vi "PH_AxisGUI_NF.panel.vi"(0 "object ref":refnum<vi>, 5 "error in (no error)":errorcluster) -> (19 "error out":errorcluster)   [LabVIEW 2014, in "PH_AxisGUI_NF.lvlib"]
doc: "By this VI a ross relais can be monitored and switched. \n\nThe indicators \"CLOSED\", \"OPEN\" and \"SWITCH STATE\" show the value of the Beckhoff-Tag: blue indicates bad tag status reference problems, darkgreen false and lightgreen on. If everything is working fine, \"CLOSED\" and \"SWITCH STATE\" should show the same value, while \"OPEN\" has the opposite value. \n\nThe oval button switches the ross relais. It should be in the same state as the \"SWITCH STATE\" indicator. \n\n\"EXIT\" closes the front panel (GUI), while \"Delete Instance\" disconnects and removes the instance from the PCS.\n\nThis VI has no machine safety relevant logig: there is neither a check of internal conclict nor with other objects, for example conflict with other ross relais. Therefore it must be handled with care and should be operated by well educated operators only. It is forseen exclusively for direct operating and testing of the system. \n\nLicense Agreement for this software:\n\nCopyright (C)\nGesellschaft für Schwerionenforschung, GSI\nPlanckstr. 1\n64291 Darmstadt\nGermany\n\nContact: D.Beck@gsi.de \n\nThis program is free software; you can redistribute it and/or modify it under the terms of the GNU General Public License as published by the Free Software Foundation; either version 2 of the license, or (at your option) any later version.\n\nThis program is distributed in the hope that it will be useful, but WITHOUT ANYW ARRANTY; without even the implied warranty of MERCHANTABILITY or FITNESS FOR A PARTICULAR PURPOSE. See the GNU General License for more details (http://www.gnu.org).\n\nGesellschaft für Schwerionenforschung, GSI\nPlanckstr. 1, 64291 Darmstadt, Germany\nFor all questions and ideas contact: M.Richter@gsi.de, H.Brand@gsi.de or D.Beck@gsi.de.\nLast update: 18-DEC-2002"
uses:
  PH_AxisGUI_NF.lvlib
  CSMotion/NF87XX/NF87XX.lvlib
  PH_Common/PH_Common.lvlib
  PH_Class/PH_Class.lvlib
panel:
  in  "Goal":string="0"
  in  "Go":bool
  in  "Reset":bool
  out "Position":i32
  out "Instance Status":u32(colorbox)
  in  "Slide 2":i32(slide) scale=-8.0..8.0
  in  "Slide 1":i32(slide) scale=-8.0..8.0
  in  "Slide 0":i32(slide) scale=-8.0..8.0
  in  "Emergeny Stop":bool
  in  "Delete":bool
  # "PCS"
  # "3.40"
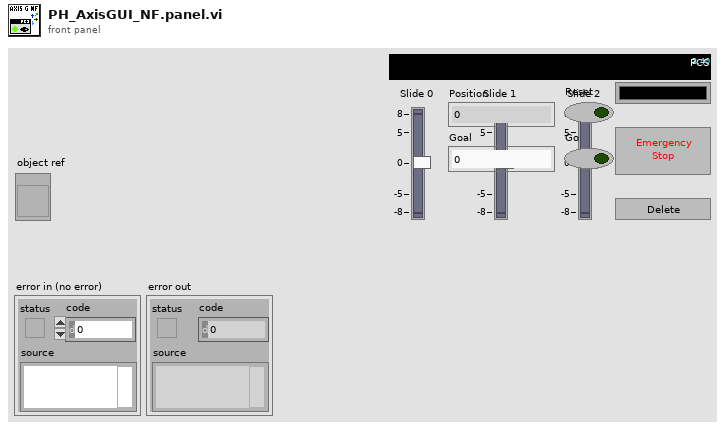
[diagram p1: front panel]
types:
  T1 = typedef "PH_AxisGUI_NF.lvlib/PH_AxisGUI_NF.i attribute.ctl" = cluster{"GUI Refs":cluster{"Delete":refnum<vi>, "Slide 0":refnum<vi>, "Slide 1":refnum<vi>, "Slide 2":refnum<vi>, "Instance Status":refnum<vi>, "Position":refnum<vi>, "Reset":refnum<vi>, "Goal":refnum<vi>, "Go":refnum<vi>}, "Instance":string, "Name Axis 0":string, "Name Axis 1":string, "Name Axis 2":string, "System":string, "Driver Type":T2, "Offset":i32, "Goal":i32}
  T2 = typedef "NF87XX.lvlib/NF87XX.driver Type.ctl" = enum16{"not defined", "3-ch open loop drv", "1-ch closed loop drv"}
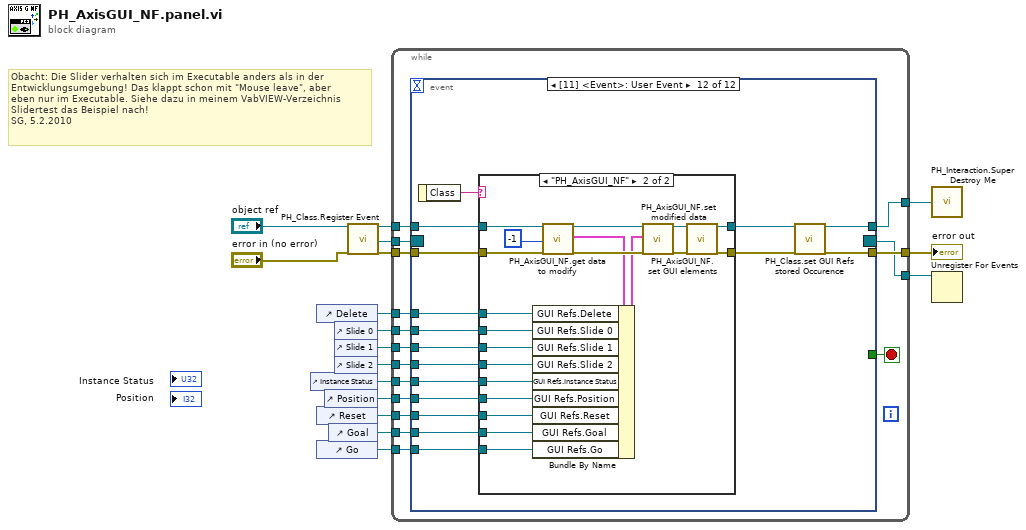
[diagram p0: block diagram]
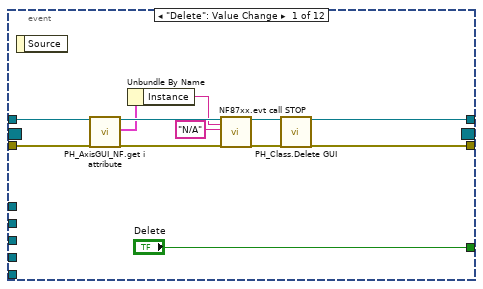
[diagram p2: hidden frame]
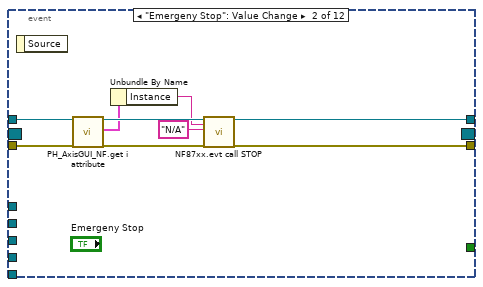
[diagram p3: hidden frame]
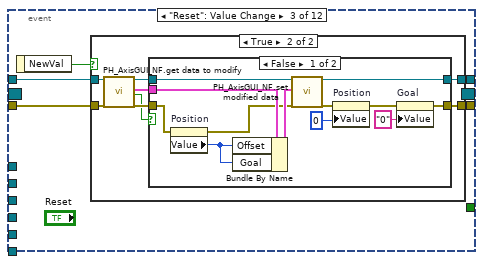
[diagram p4: hidden frame]
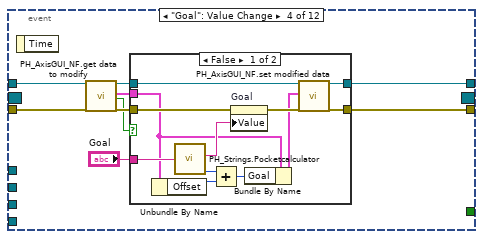
[diagram p7: hidden frame]
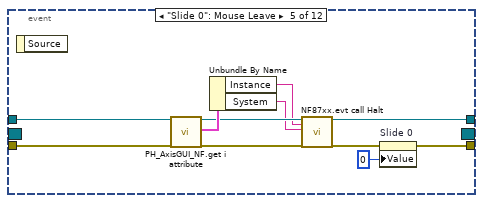
[diagram p9: hidden frame]
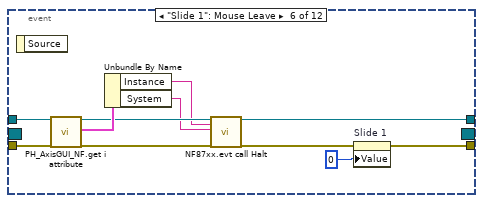
[diagram p10: hidden frame]
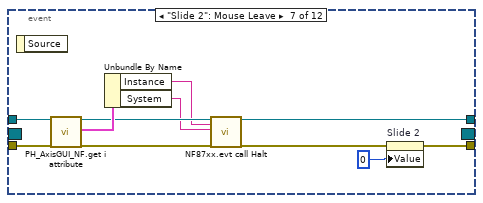
[diagram p11: hidden frame]
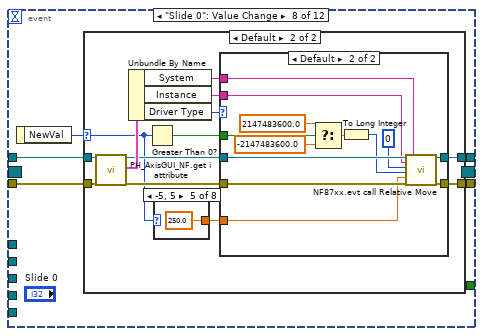
[diagram p12: hidden frame]
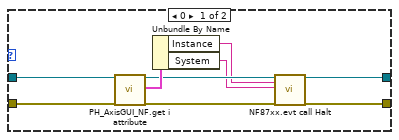
[diagram p13: hidden frame]
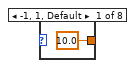
[diagram p14: hidden frame]
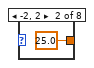
[diagram p15: hidden frame]
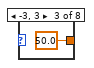
[diagram p16: hidden frame]
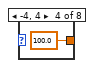
[diagram p17: hidden frame]
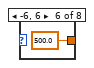
[diagram p18: hidden frame]
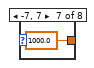
[diagram p19: hidden frame]
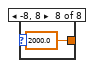
[diagram p20: hidden frame]
diagram:
  # "Obacht: Die Slider verhalten sich im Executable anders als in der\nEntwicklungsumgebung! Das klappt schon mit \"Mouse leave\", aber \neben nur im Executable. Siehe dazu in meinem VabVIEW-Verzeichnis\nSlidertest das Beispiel nach!\nSG, 5.2.2010"
  n1 = control-ref of="Instance Status"() -> (w7:refnum<vi>)
  n2 = control-ref of="Delete"() -> (w11:refnum<vi>)
  n3 = control-ref of="Reset"() -> (w5:refnum<vi>)
  n4 = control-ref of="Go"() -> (w3:refnum<vi>)
  n5 = control-ref of="Position"() -> (w6:refnum<vi>)
  n6 = control-ref of="Goal"() -> (w4:refnum<vi>)
  n7 = control-ref of="Slide 0"() -> (w10:refnum<vi>)
  n8 = control-ref of="Slide 1"() -> (w9:refnum<vi>)
  n9 = control-ref of="Slide 2"() -> (w8:refnum<vi>)
  n10 = call "PH_Class.Register Event.vi"("i ref in"="object ref", "error in (no error)"="error in (no error)") -> ("i ref out"=w15:refnum<vi>, "Event Registration Refnum"=w13:refnum<event-registration>, "error out"=w14:errorcluster)  [unwired: 15 in]
  n11 = while {
    tunnel: w15 -> [w30]
    tunnel: [w29] -> w17
    tunnel: w14 -> [w32]
    tunnel: [w31] -> w16
    tunnel: w13 -> [w28]
    tunnel: [w27] -> w12
    tunnel: w11 -> [w26]
    tunnel: w10 -> [w25]
    tunnel: w9 -> [w24]
    tunnel: w8 -> [w23]
    tunnel: w7 -> [w22]
    tunnel: w6 -> [w21]
    tunnel: w5 -> [w20]
    tunnel: w4 -> [w19]
    tunnel: w3 -> [w18]
    stop <- w33 stop-if-true
    n12 = event shown="[11] <Event>: User Event" {
      selector: w28 -> [_ _ _ _ _ _ _ _ _ _ _ _]
      dyn-events: [_ _ _ _ _ _ _ _ _ _ _ _] -> w27
      timeout: _ -> [_ _ _ _ _ _ _ _ _ _ _ _]
      tunnel: ["Delete" _ _ _ _ _ _ _ _ _ _ _] -> w33
      tunnel: w30 -> [w39 w50 w57 w87 w112 w126 w137 w142 w200 w249 w299 w357]
      tunnel: w32 -> [w37 w52 w56 w90 w110 w124 w135 w144 w199 w250 w300 w356]
      tunnel: [w34 w54 w59 w88 w116 w120 w131 w143 w197 w247 w298 w359] -> w31
      tunnel: [w35 w53 w58 w86 w113 w127 w138 w141 w198 w246 w297 w360] -> w29
      tunnel: w26 -> [_ _ _ _ _ _ _ _ _ _ _ w353]
      tunnel: w25 -> [_ _ _ _ _ _ _ _ _ _ _ w352]
      tunnel: w24 -> [_ _ _ _ _ _ _ _ _ _ _ w351]
      tunnel: w23 -> [_ _ _ _ _ _ _ _ _ _ _ w350]
      tunnel: w22 -> [_ _ _ _ _ _ _ _ _ _ _ w349]
      tunnel: w21 -> [_ _ _ _ _ _ _ _ _ _ _ w348]
      tunnel: w20 -> [_ _ _ _ _ _ _ _ _ _ _ w347]
      tunnel: w19 -> [_ _ _ _ _ _ _ _ _ _ _ w346]
      tunnel: w18 -> [_ _ _ _ _ _ _ _ _ _ _ w345]
      event "Delete": Value Change {
        n13 = event-data() -> ()  [unwired: 1 in, 1 out]
        n14 = call "PH_AxisGUI_NF.get i attribute.vi"("i ref in"=w39, "error in (no error)"=w37) -> ("i ref out"=w43:refnum<vi>, "i attribute"=w42:T1, "error out"=w44:errorcluster)  [unwired: 15 in]
        n15 = Unbundle By Name(w42) -> ("Instance"=w41:string)
        n16 = call "NF87xx.evt call STOP.vi"("i ref in"=w43, "Instance"=w41, "System (N/A)"="N/A", "error in (no error)"=w44) -> ("i ref out"=w38:refnum<vi>, "error out"=w36:errorcluster)  [unwired: 14 in]
        n17 = call "PH_Class.Delete GUI.vi"("VI in"=w38, "error in (no error)"=w36) -> ("VI out"=w35:refnum<vi>, "error out"=w34:errorcluster)  [unwired: 16 in]
      }
      event "Emergeny Stop": Value Change {
        n18 = event-data() -> ()  [unwired: 1 in, 1 out]
        n19 = call "PH_AxisGUI_NF.get i attribute.vi"("i ref in"=w50, "error in (no error)"=w52) -> ("i ref out"=w49:refnum<vi>, "i attribute"=w48:T1, "error out"=w51:errorcluster)  [unwired: 15 in]
        n20 = Unbundle By Name(w48) -> ("Instance"=w47:string)
        n21 = call "NF87xx.evt call STOP.vi"("i ref in"=w49, "Instance"=w47, "System (N/A)"="N/A", "error in (no error)"=w51) -> ("i ref out"=w53:refnum<vi>, "error out"=w54:errorcluster)  [unwired: 14 in]
      }
      event "Reset": Value Change {
        n22 = event-data() -> ("NewVal"=w55:bool)  [unwired: 1 in]
        n23 = case shown="True" w55 {
          tunnel: [w60 w69] -> w59
          tunnel: [w61 w68] -> w58
          tunnel: w57 -> [w61 w67]
          tunnel: w56 -> [w60 w65]
          frame False {
          }
          frame True {
            n24 = call "PH_AxisGUI_NF.get data to modify.vi"("i ref in"=w67, "error in (no error)"=w65) -> ("i ref out"=w66:refnum<vi>, "i attribute"=w62:T1, "timed out"=w63:bool, "error out"=w64:errorcluster)  [unwired: 14 in]
            n25 = case shown="False" w63 {
              tunnel: [w72 w82] -> w69
              tunnel: [w81 w83] -> w68
              tunnel: w66 -> [w80 w83]
              tunnel: w64 -> [w77 w82]
              tunnel: w62 -> [w79 _]
              frame False {
                n26 = property on="Position" class="DigNum (strict)"(error in=w77) -> (error out=w76:errorcluster, "Value"=w70:i32)  [unwired: 1 in, 1 out]
                n27 = Bundle By Name(cluster=w79, "Offset"=w70, "Goal"=w70) -> (w78:T1)
                n28 = call "PH_AxisGUI_NF.set modified data.vi"("i ref in"=w80, "i attribute"=w78, "error in (no error)"=w76) -> ("i ref out"=w81:refnum<vi>, "error out"=w75:errorcluster)  [unwired: 15 in]
                n29 = property on="Position" class="DigNum (strict)"(error in=w75, "Value"=0 ("Position")) -> (error out=w73:errorcluster)  [unwired: 1 in, 1 out]
                n30 = property on="Goal" class="Str"(error in=w73, "Value"="0" ("Goal")) -> (error out=w72:errorcluster)  [unwired: 1 in, 1 out]
              }
              frame True {
              }
            }
          }
        }
      }
      event "Goal": Value Change {
        n31 = event-data() -> ()  [unwired: 1 in, 1 out]
        n32 = call "PH_AxisGUI_NF.get data to modify.vi"("i ref in"=w87, "error in (no error)"=w90) -> ("i ref out"=w91:refnum<vi>, "i attribute"=w85:T1, "timed out"=w84:bool, "error out"=w89:errorcluster)  [unwired: 14 in]
        n33 = case shown="False" w84 {
          tunnel: "Goal" -> [w104 _]
          tunnel: w91 -> [w102 w106]
          tunnel: w89 -> [w101 w105]
          tunnel: [w99 w105] -> w88
          tunnel: [w98 w106] -> w86
          tunnel: w85 -> [w96 _]
          frame False {
            n34 = Unbundle By Name(w96) -> ("Offset"=w94:i32)
            n35 = call "PH_Strings.Pocketcalculator.vi"("Input"=w104) -> ("String Integer"=w103:string, "Integer"=w95:i32)  [unwired: 2 out]
            n36 = Add(x=w95, y=w94) -> (x+y=w93:i32)
            n37 = property on="Goal" class="Str"(error in=w101, "Value"=w103) -> (error out=w100:errorcluster)  [unwired: 1 in, 1 out]
            n38 = Bundle By Name(cluster=w96, "Goal"=w93) -> (w97:T1)
            n39 = call "PH_AxisGUI_NF.set modified data.vi"("i ref in"=w102, "i attribute"=w97, "error in (no error)"=w100) -> ("i ref out"=w98:refnum<vi>, "error out"=w99:errorcluster)  [unwired: 15 in]
          }
          frame True {
          }
        }
      }
      event "Slide 0": Mouse Leave {
        n40 = event-data() -> ()  [unwired: 1 in, 1 out]
        n41 = call "PH_AxisGUI_NF.get i attribute.vi"("i ref in"=w112, "error in (no error)"=w110) -> ("i ref out"=w111:refnum<vi>, "i attribute"=w115:T1, "error out"=w109:errorcluster)  [unwired: 15 in]
        n42 = Unbundle By Name(w115) -> ("Instance"=w108:string, "System"=w107:string)
        n43 = call "NF87xx.evt call Halt.vi"("i ref in"=w111, "Instance"=w108, "System"=w107, "error in (no error)"=w109) -> ("i ref out"=w113:refnum<vi>, "error out"=w114:errorcluster)  [unwired: 14 in]
        n44 = property on="Slide 0" class="Slide (strict)"(error in=w114, "Value"=0 ("Slide 0")) -> (error out=w116:errorcluster)  [unwired: 1 in, 1 out]
      }
      event "Slide 1": Mouse Leave {
        n45 = event-data() -> ()  [unwired: 1 in, 1 out]
        n46 = call "PH_AxisGUI_NF.get i attribute.vi"("i ref in"=w126, "error in (no error)"=w124) -> ("i ref out"=w125:refnum<vi>, "i attribute"=w128:T1, "error out"=w123:errorcluster)  [unwired: 15 in]
        n47 = Unbundle By Name(w128) -> ("Instance"=w122:string, "System"=w118:string)
        n48 = call "NF87xx.evt call Halt.vi"("i ref in"=w125, "Instance"=w122, "System"=w118, "error in (no error)"=w123) -> ("i ref out"=w127:refnum<vi>, "error out"=w121:errorcluster)  [unwired: 14 in]
        n49 = property on="Slide 1" class="Slide (strict)"(error in=w121, "Value"=0 ("Slide 0")) -> (error out=w120:errorcluster)  [unwired: 1 in, 1 out]
      }
      event "Slide 2": Mouse Leave {
        n50 = event-data() -> ()  [unwired: 1 in, 1 out]
        n51 = call "PH_AxisGUI_NF.get i attribute.vi"("i ref in"=w137, "error in (no error)"=w135) -> ("i ref out"=w136:refnum<vi>, "i attribute"=w139:T1, "error out"=w134:errorcluster)  [unwired: 15 in]
        n52 = Unbundle By Name(w139) -> ("Instance"=w133:string, "System"=w129:string)
        n53 = call "NF87xx.evt call Halt.vi"("i ref in"=w136, "Instance"=w133, "System"=w129, "error in (no error)"=w134) -> ("i ref out"=w138:refnum<vi>, "error out"=w132:errorcluster)  [unwired: 14 in]
        n54 = property on="Slide 2" class="Slide (strict)"(error in=w132, "Value"=0 ("Slide 0")) -> (error out=w131:errorcluster)  [unwired: 1 in, 1 out]
      }
      event "Slide 0": Value Change {
        n55 = event-data() -> ("NewVal"=w140:i32)  [unwired: 1 in]
        n56 = case shown="Default" w140 {
          selector: w140 -> [_ w155]
          tunnel: w144 -> [w147 w165]
          tunnel: [w146 w163] -> w143
          tunnel: w142 -> [w149 w162]
          tunnel: [w148 w160] -> w141
          frame 0 {
            n57 = call "PH_AxisGUI_NF.get i attribute.vi"("i ref in"=w149, "error in (no error)"=w147) -> ("i ref out"=w152:refnum<vi>, "i attribute"=w153:T1, "error out"=w151:errorcluster)  [unwired: 15 in]
            n58 = Unbundle By Name(w153) -> ("Instance"=w150:string, "System"=w145:string)
            n59 = call "NF87xx.evt call Halt.vi"("i ref in"=w152, "Instance"=w150, "System"=w145, "error in (no error)"=w151) -> ("i ref out"=w148:refnum<vi>, "error out"=w146:errorcluster)  [unwired: 14 in]
          }
          frame Default {
            n60 = call "PH_AxisGUI_NF.get i attribute.vi"("i ref in"=w162, "error in (no error)"=w165) -> ("i ref out"=w161:refnum<vi>, "i attribute"=w166:T1, "error out"=w164:errorcluster)  [unwired: 15 in]
            n61 = Unbundle By Name(w166) -> ("System"=w157:string, "Instance"=w159:string, "Driver Type"=w156:T2)
            n62 = Greater Than 0?(x=w155) -> (x > 0?=w158:bool)
            n63 = case shown="-5, 5" w155 {
              tunnel: [10.0 ("velocity (10 .. 2000)") 25.0 ("velocity (10 .. 2000)") 50.0 ("velocity (10 .. 2000)") 100.0 ("velocity (10 .. 2000)") 250.0 ("velocity (10 .. 2000)") 500.0 ("velocity (10 .. 2000)") 1000.0 ("velocity (10 .. 2000)") 2000.0 ("velocity (10 .. 2000)")] -> w154
              frame -1, 1, Default {
              }
              frame -2, 2 {
              }
              frame -3, 3 {
              }
              frame -4, 4 {
              }
              frame -5, 5 {
              }
              frame -6, 6 {
              }
              frame -7, 7 {
              }
              frame -8, 8 {
              }
            }
            n64 = case shown="Default" w156 {
              tunnel: w164 -> [w180 w195]
              tunnel: [w179 w194] -> w163
              tunnel: w161 -> [w182 w193]
              tunnel: [w181 w192] -> w160
              tunnel: w159 -> [w176 w191]
              tunnel: w158 -> [w177 w189]
              tunnel: w157 -> [w175 w184]
              tunnel: w154 -> [w178 w183]
              frame "1-ch closed loop drv" {
                n65 = call "NF87xx.evt call Absolute Move.vi"("i ref in"=w182, "Instance"=w176, "forward?"=w177, "velocity (10 .. 2000)"=w178, "error in (no error)"=w180, "System"=w175) -> ("i ref out"=w181:refnum<vi>, "error out"=w179:errorcluster)  [unwired: 12 in]
              }
              frame Default {
                n66 = Select(t=2147483600.0, s=w189, f=-2147483600.0) -> (s? t:f=w185:dbl)
                n67 = To Long Integer(number=w185) -> (32bit integer=w188:i32)
                n68 = call "NF87xx.evt call Relative Move.vi"("i ref in"=w193, "Instance"=w191, "Motor (0, 1 or 2)"=0, "steps"=w188, "velocity (10 .. 2000)"=w183, "error in (no error)"=w195, "System"=w184) -> ("i ref out"=w192:refnum<vi>, "error out"=w194:errorcluster)  [unwired: 11 in]
              }
            }
          }
        }
      }
      event "Slide 1": Value Change {
        n69 = event-data() -> ("NewVal"=w196:i32)  [unwired: 1 in]
        n70 = case shown="Default" w196 {
          selector: w196 -> [_ w211]
          tunnel: w199 -> [w203 w221]
          tunnel: [w202 w219] -> w197
          tunnel: w200 -> [w205 w218]
          tunnel: [w204 w216] -> w198
          frame 0 {
            n71 = call "PH_AxisGUI_NF.get i attribute.vi"("i ref in"=w205, "error in (no error)"=w203) -> ("i ref out"=w208:refnum<vi>, "i attribute"=w209:T1, "error out"=w207:errorcluster)  [unwired: 15 in]
            n72 = Unbundle By Name(w209) -> ("Instance"=w206:string, "System"=w201:string)
            n73 = call "NF87xx.evt call Halt.vi"("i ref in"=w208, "Instance"=w206, "System"=w201, "error in (no error)"=w207) -> ("i ref out"=w204:refnum<vi>, "error out"=w202:errorcluster)  [unwired: 14 in]
          }
          frame Default {
            n74 = call "PH_AxisGUI_NF.get i attribute.vi"("i ref in"=w218, "error in (no error)"=w221) -> ("i ref out"=w217:refnum<vi>, "i attribute"=w222:T1, "error out"=w220:errorcluster)  [unwired: 15 in]
            n75 = Unbundle By Name(w222) -> ("System"=w213:string, "Instance"=w215:string, "Driver Type"=w212:T2)
            n76 = Greater Than 0?(x=w211) -> (x > 0?=w214:bool)
            n77 = case shown="-1, 1, Default" w211 {
              tunnel: [10.0 ("velocity (10 .. 2000)") 25.0 ("velocity (10 .. 2000)") 50.0 ("velocity (10 .. 2000)") 100.0 ("velocity (10 .. 2000)") 250.0 ("velocity (10 .. 2000)") 500.0 ("velocity (10 .. 2000)") 1000.0 ("velocity (10 .. 2000)") 2000.0 ("velocity (10 .. 2000)")] -> w210
              frame -1, 1, Default {
              }
              frame -2, 2 {
              }
              frame -3, 3 {
              }
              frame -4, 4 {
              }
              frame -5, 5 {
              }
              frame -6, 6 {
              }
              frame -7, 7 {
              }
              frame -8, 8 {
              }
            }
            n78 = case shown="Default" w212 {
              tunnel: w220 -> [w231 w245]
              tunnel: [w231 w244] -> w219
              tunnel: w217 -> [w232 w243]
              tunnel: [w232 w242] -> w216
              tunnel: w215 -> [_ w241]
              tunnel: w214 -> [_ w239]
              tunnel: w210 -> [_ w233]
              tunnel: w213 -> [_ w234]
              frame "1-ch closed loop drv" {
              }
              frame Default {
                n79 = Select(t=2147483600.0, s=w239, f=-2147483600.0) -> (s? t:f=w235:dbl)
                n80 = To Long Integer(number=w235) -> (32bit integer=w238:i32)
                n81 = call "NF87xx.evt call Relative Move.vi"("i ref in"=w243, "Instance"=w241, "Motor (0, 1 or 2)"=1, "steps"=w238, "velocity (10 .. 2000)"=w233, "error in (no error)"=w245, "System"=w234) -> ("i ref out"=w242:refnum<vi>, "error out"=w244:errorcluster)  [unwired: 11 in]
              }
            }
          }
        }
      }
      event "Slide 2": Value Change {
        n82 = event-data() -> ("NewVal"=w248:i32)  [unwired: 1 in]
        n83 = case shown="Default" w248 {
          selector: w248 -> [_ w261]
          tunnel: w250 -> [w253 w271]
          tunnel: [w252 w269] -> w247
          tunnel: w249 -> [w255 w268]
          tunnel: [w254 w266] -> w246
          frame 0 {
            n84 = call "PH_AxisGUI_NF.get i attribute.vi"("i ref in"=w255, "error in (no error)"=w253) -> ("i ref out"=w258:refnum<vi>, "i attribute"=w259:T1, "error out"=w257:errorcluster)  [unwired: 15 in]
            n85 = Unbundle By Name(w259) -> ("Instance"=w256:string, "System"=w251:string)
            n86 = call "NF87xx.evt call Halt.vi"("i ref in"=w258, "Instance"=w256, "System"=w251, "error in (no error)"=w257) -> ("i ref out"=w254:refnum<vi>, "error out"=w252:errorcluster)  [unwired: 14 in]
          }
          frame Default {
            n87 = call "PH_AxisGUI_NF.get i attribute.vi"("i ref in"=w268, "error in (no error)"=w271) -> ("i ref out"=w267:refnum<vi>, "i attribute"=w272:T1, "error out"=w270:errorcluster)  [unwired: 15 in]
            n88 = Unbundle By Name(w272) -> ("System"=w263:string, "Instance"=w265:string, "Driver Type"=w262:T2)
            n89 = Greater Than 0?(x=w261) -> (x > 0?=w264:bool)
            n90 = case shown="-1, 1, Default" w261 {
              tunnel: [10.0 ("velocity (10 .. 2000)") 25.0 ("velocity (10 .. 2000)") 50.0 ("velocity (10 .. 2000)") 100.0 ("velocity (10 .. 2000)") 250.0 ("velocity (10 .. 2000)") 500.0 ("velocity (10 .. 2000)") 1000.0 ("velocity (10 .. 2000)") 2000.0 ("velocity (10 .. 2000)")] -> w260
              frame -1, 1, Default {
              }
              frame -2, 2 {
              }
              frame -3, 3 {
              }
              frame -4, 4 {
              }
              frame -5, 5 {
              }
              frame -6, 6 {
              }
              frame -7, 7 {
              }
              frame -8, 8 {
              }
            }
            n91 = case shown="Default" w262 {
              tunnel: w270 -> [w293 w294]
              tunnel: [w292 w294] -> w269
              tunnel: w267 -> [w291 w295]
              tunnel: [w290 w295] -> w266
              tunnel: w265 -> [w289 _]
              tunnel: w264 -> [w287 _]
              tunnel: w263 -> [w282 _]
              tunnel: w260 -> [w281 _]
              frame Default {
                n92 = Select(t=2147483600.0, s=w287, f=-2147483600.0) -> (s? t:f=w283:dbl)
                n93 = To Long Integer(number=w283) -> (32bit integer=w286:i32)
                n94 = call "NF87xx.evt call Relative Move.vi"("i ref in"=w291, "Instance"=w289, "Motor (0, 1 or 2)"=2, "steps"=w286, "velocity (10 .. 2000)"=w281, "error in (no error)"=w293, "System"=w282) -> ("i ref out"=w290:refnum<vi>, "error out"=w292:errorcluster)  [unwired: 11 in]
              }
              frame "1-ch closed loop drv" {
              }
            }
          }
        }
      }
      event "Go": Value Change {
        n95 = event-data() -> ("NewVal"=w296:bool)  [unwired: 1 in]
        n96 = case shown="True" w296 {
          tunnel: w300 -> [w301 w312]
          tunnel: [w301 w310] -> w298
          tunnel: w299 -> [w302 w309]
          tunnel: [w302 w307] -> w297
          frame False {
          }
          frame True {
            n97 = call "PH_AxisGUI_NF.get i attribute.vi"("i ref in"=w309, "error in (no error)"=w312) -> ("i ref out"=w308:refnum<vi>, "i attribute"=w313:T1, "error out"=w311:errorcluster)  [unwired: 15 in]
            n98 = Unbundle By Name(w313) -> ("Driver Type"=w304:T2, "System"=w305:string, "Instance"=w306:string, "Goal"=w303:i32)
            n99 = case shown="\"1-ch closed loop drv\"" w304 {
              tunnel: w311 -> [w324 w343]
              tunnel: [w322 w343] -> w310
              tunnel: w308 -> [w323 w344]
              tunnel: [w321 w344] -> w307
              tunnel: w306 -> [w315 _]
              tunnel: w305 -> [w316 _]
              tunnel: w303 -> [w314 _]
              frame "1-ch closed loop drv" {
                n100 = flat-sequence {
                  tunnel: w324 -> [w331]
                  tunnel: w323 -> [w330]
                  tunnel: w316 -> [w329]
                  tunnel: w315 -> [w328]
                  tunnel: [w326] -> w320
                  tunnel: [w325] -> w319
                  tunnel: w320 -> [w334]
                  tunnel: w319 -> [w333]
                  tunnel: [w334] -> w318
                  tunnel: [w333] -> w317
                  tunnel: [w341] -> w321
                  tunnel: [w339] -> w322
                  tunnel: w318 -> [w340]
                  tunnel: w317 -> [w342]
                  tunnel: w316 -> [w337]
                  tunnel: w315 -> [w336]
                  tunnel: w314 -> [w335]
                  frame #0 {
                    n101 = call "NF87xx.evt call Set Velocity.vi"("i ref in"=w330, "Instance"=w328, "velocity (0 .. 2000)"=2000.0 ("velocity (10 .. 2000)"), "error in (no error)"=w331, "System"=w329) -> ("i ref out"=w325:refnum<vi>, "error out"=w326:errorcluster)  [unwired: 13 in]
                  }
                  frame #1 {
                    n102 = Wait (ms)(milliseconds to wait=u32 200) -> ()  [unwired: 1 out]
                  }
                  frame #2 {
                    n103 = call "NF87xx.evt call Move 2 Pos.vi"("i ref in"=w342, "Instance"=w336, "Position"=w335, "Immediately?"=TRUE, "error in (no error)"=w340, "System"=w337) -> ("i ref out"=w341:refnum<vi>, "error out"=w339:errorcluster)  [unwired: 12 in]
                  }
                }
              }
              frame Default {
              }
            }
          }
        }
      }
      event User Event {
        n104 = event-data() -> ("Class"=w354:string)  [unwired: 1 in]
        n105 = case shown="\"PH_AxisGUI_NF\"" w354 {
          tunnel: [w362 w382] -> w358
          tunnel: w357 -> [w362 w377]
          tunnel: w356 -> [w361 w375]
          tunnel: [w361 w372] -> w355
          tunnel: w353 -> [_ w371]
          tunnel: w352 -> [_ w370]
          tunnel: w351 -> [_ w369]
          tunnel: w350 -> [_ w368]
          tunnel: w349 -> [_ w367]
          tunnel: w348 -> [_ w366]
          tunnel: w347 -> [_ w365]
          tunnel: w346 -> [_ w364]
          tunnel: w345 -> [_ w363]
          frame Default {
          }
          frame "PH_AxisGUI_NF" {
            n106 = call "PH_AxisGUI_NF.get data to modify.vi"("i ref in"=w377, "ms timeout (10000)"=-1, "error in (no error)"=w375) -> ("i ref out"=w381:refnum<vi>, "i attribute"=w379:T1, "error out"=w380:errorcluster)  [unwired: 13 in, 1 out]
            n107 = Bundle By Name(cluster=w379, "GUI Refs.Delete"=w371, "GUI Refs.Slide 0"=w370, "GUI Refs.Slide 1"=w369, "GUI Refs.Slide 2"=w368, "GUI Refs.Instance Status"=w367, "GUI Refs.Position"=w366, "GUI Refs.Reset"=w365, "GUI Refs.Goal"=w364, "GUI Refs.Go"=w363) -> (w378:T1)
            n108 = call "PH_AxisGUI_NF.set modified data.vi"("i ref in"=w381, "i attribute"=w378, "error in (no error)"=w380) -> ("i ref out"=w376:refnum<vi>, "error out"=w374:errorcluster)  [unwired: 15 in]
            n109 = call "PH_AxisGUI_NF.set GUI elements.vi"("i ref in"=w376, "error in (no error)"=w374) -> ("i ref out"=w382:refnum<vi>, "error out"=w372:errorcluster)  [unwired: 16 in]
          }
        }
        n110 = call "PH_Class.set GUI Refs stored Occurence.vi"("i ref in"=w358, "error in (no error)"=w355) -> ("i ref out"=w360:refnum<vi>, "error out"=w359:errorcluster)  [unwired: 16 in]
      }
    }
  }
  "error out" <- w16
  n111 = call "PH_Interaction.Super Destroy Me.vi"("i ref out"=w17) -> ()
  n112 = Unregister For Events(event registration refnum=w12) -> ()  [unwired: 1 in, 1 out]
